vi "Build DashBoard Data.vi"() -> ()   [LabVIEW 2011]
doc: "This VI builds data and sends it back to the dashboard PC program. By default it sends back the raw values for the first analog, digital, and solenoid module. Modify it to send back the data you want to view. Consider adding higher level data to the Dashboard Datatype.ctl and to this VI. Then update the Dashboard to display the data however you like.\n\nThis software is licensed. Open the labview\\readme\\WPI Robotics Library Open Source License.txt file for more information."
uses:
  hiPri Dashboard Datatype.ctl
  Dashboard Datatype.ctl
  Robot Global Data.vi
panel:
  in  "Dashboard Data":T1={"Bridge Balance"=FALSE, "Gyro"=0.0, "Left Drive"=0.0, "Right Drive"=0.0, "Shooter Ready"=FALSE, "Compass"=0.0, "Turret Enc"=0.0, "Gear"=0, "Turret Postion"=1.0, "Turret Bump"=FALSE, "Collector System Enabled?"=FALSE, "Personality"="", "Brake"=FALSE} {"Gear" items=["HIGH", "LOW"]; "Compass" scale=0.0..-180.0; "Gyro" scale=-180.0..180.0}
  in  "HiPri":T2
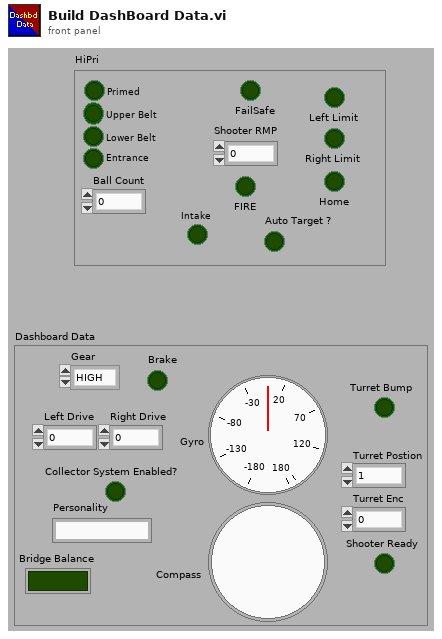
[diagram p1: front panel]
types:
  T1 = typedef "Dashboard Datatype.ctl" = cluster{"Bridge Balance":bool, "Gyro":dbl, "Left Drive":dbl, "Right Drive":dbl, "Shooter Ready":bool, "Compass":dbl, "Turret Enc":dbl, "Gear":u16, "Turret Postion":dbl, "Turret Bump":bool, "Collector System Enabled?":bool, "Personality":string, "Brake":bool}
  T2 = typedef "hiPri Dashboard Datatype.ctl" = cluster{"Ball Count":dbl, "Shooter RMP":dbl, "FIRE":bool, "FailSafe":bool, "Entrance":bool, "Lower Belt":bool, "Upper Belt":bool, "Primed":bool, "Intake":bool, "Right Limit":bool, "Home":bool, "Left Limit":bool, "Auto Target ?":bool}
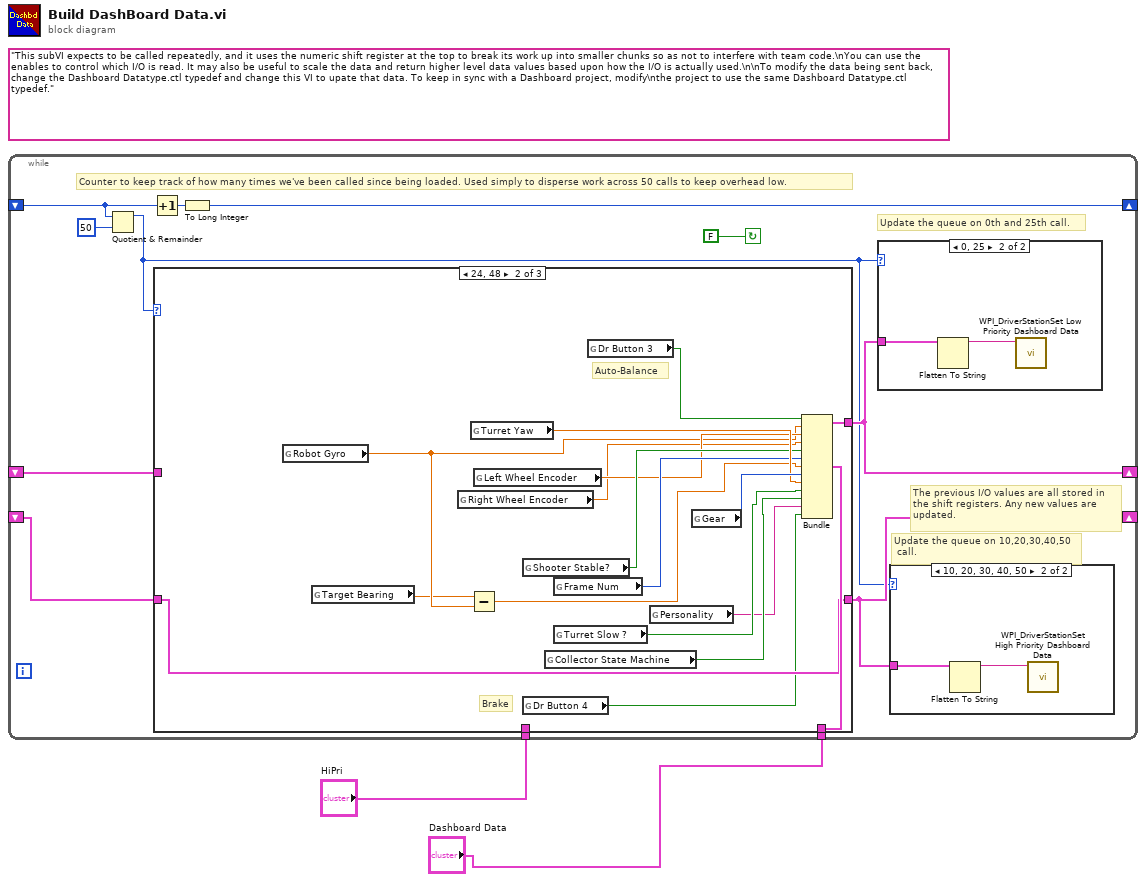
[diagram p0: block diagram]
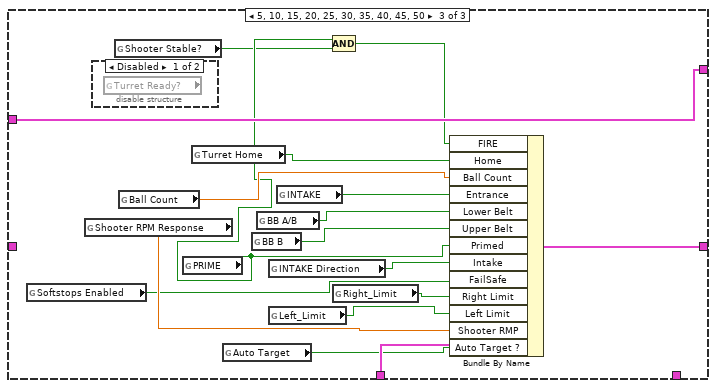
[diagram p5: hidden frame]
diagram:
  (unwired) "This subVI expects to be called repeatedly, and it uses the numeric shift register at the top to break its work up into smaller chunks so as not to interfere with team code.\nYou can use the enables to control which I/O is read. It may also be useful to scale the data and return higher level data values based upon how the I/O is actually used.\n\nTo modify the data being sent back, change the Dashboard Datatype.ctl typedef and change this VI to upate that data. To keep in sync with a Dashboard project, modify\nthe project to use the same Dashboard Datatype.ctl typedef."
  n1 = while {
    shift-right: [w9] -> _
    shift-left: _ -> [w10]
    shift-right: [w7] -> _
    shift-left: _ -> [w12]
    tunnel: "Dashboard Data" -> [w8]
    tunnel: "HiPri" -> [w6]
    shift-right: [w5] -> _
    shift-left: _ -> [w4]
    stop <- FALSE continue-if-true
    # "Update the queue on 10,20,30,40,50\n call."
    # "Counter to keep track of how many times we've been called since being loaded. Used simply to disperse work across 50 calls to keep overhead low."
    # "Update the queue on 0th and 25th call."
    # "The previous I/O values are all stored in\nthe shift registers. Any new values are\nupdated."
    n2 = Quotient & Remainder(x=w10, y=50) -> (x-y*floor(x/y)=w3:i32)  [unwired: 1 out]
    n3 = Increment(x=w10) -> (x+1=w14:i32)
    n4 = case shown="24, 48" w3 {
      tunnel: [w20 w36 w54] -> w7
      tunnel: w12 -> [w20 _ w54]
      tunnel: w8 -> [_ w37 _]
      tunnel: w6 -> [_ _ w53]
      tunnel: [w19 w35 w52] -> w5
      tunnel: w4 -> [w19 w35 _]
      frame Default {
        # "Don't update any I/O"
      }
      frame 24, 48 {
        # "Brake"
        # "Auto-Balance"
        n5 = global read "Robot Global Data.vi" "Robot Gyro"() -> (w26:dbl)
        n6 = global read "Robot Global Data.vi" "Target Bearing"() -> (w25:dbl)
        n7 = global read "Robot Global Data.vi" "Right Wheel Encoder"() -> (w29:dbl)
        n8 = Subtract(x=w25, y=w26) -> (x-y=w24:dbl)
        n9 = global read "Robot Global Data.vi" "Turret Yaw"() -> (w33:dbl)
        n10 = global read "Robot Global Data.vi" "Left Wheel Encoder"() -> (w30:dbl)
        n11 = global read "Robot Global Data.vi" "Shooter Stable?"() -> (w31:bool)
        n12 = global read "Robot Global Data.vi" "Dr Button 4"() -> (w21:bool)
        n13 = global read "Robot Global Data.vi" "Collector State Machine"() -> (w27:bool)
        n14 = global read "Robot Global Data.vi" "Frame Num"() -> (w32:i32)
        n15 = global read "Robot Global Data.vi" "Turret Slow ?"() -> (w28:bool)
        n16 = global read "Robot Global Data.vi" "Dr Button 3"() -> (w22:bool)
        n17 = global read "Robot Global Data.vi" "Personality"() -> (w23:string)
        n18 = global read "Robot Global Data.vi" "Gear"() -> (w34:u16)
        n19 = Bundle(cluster=w37, "Bridge Balance"=w22, "Gyro"=w26, "Left Drive"=w30, "Right Drive"=w29, "Shooter Ready"=w31, "Compass"=w32, "Turret Enc"=w24, "Gear"=w34, "Turret Postion"=w33, "Turret Bump"=w28, "Collector System Enabled?"=w27, "Personality"=w23, "Brake"=w21) -> (w36:T1)
      }
      frame 5, 10, 15, 20, 25, 30, 35, 40, 45, 50 {
        n20 = global read "Robot Global Data.vi" "Softstops Enabled"() -> (w45:bool)
        n21 = global read "Robot Global Data.vi" "Shooter RPM Response"() -> (w50:dbl)
        n22 = disable-structure shown="Disabled" {
          frame Disabled {
            n23 = global read "Robot Global Data.vi" "Turret Ready?"() -> ()  [unwired: 1 out]
          }
          frame Enabled {
          }
        }
        n24 = global read "Robot Global Data.vi" "Shooter Stable?"() -> (w38:bool)
        n25 = global read "Robot Global Data.vi" "Ball Count"() -> (w49:dbl)
        n26 = global read "Robot Global Data.vi" "PRIME"() -> (w43:bool)
        n27 = global read "Robot Global Data.vi" "Turret Home"() -> (w51:bool)
        n28 = global read "Robot Global Data.vi" "Auto Target"() -> (w39:bool)
        n29 = global read "Robot Global Data.vi" "BB B"() -> (w46:bool)
        n30 = global read "Robot Global Data.vi" "BB A/B"() -> (w47:bool)
        n31 = global read "Robot Global Data.vi" "INTAKE Direction"() -> (w44:bool)
        n32 = global read "Robot Global Data.vi" "Left_Limit"() -> (w40:bool)
        n33 = global read "Robot Global Data.vi" "INTAKE"() -> (w48:bool)
        n34 = Compound Arithmetic op=AND(w43, w38) -> (w42:bool)
        n35 = global read "Robot Global Data.vi" "Right_Limit"() -> (w41:bool)
        n36 = Bundle By Name(cluster=w53, "FIRE"=w42, "Home"=w51, "Ball Count"=w49, "Entrance"=w48, "Lower Belt"=w47, "Upper Belt"=w46, "Primed"=w43, "Intake"=w44, "FailSafe"=w45, "Right Limit"=w41, "Left Limit"=w40, "Shooter RMP"=w50, "Auto Target ?"=w39) -> (w52:T2)
      }
    }
    n37 = To Long Integer(number=w14) -> (32bit integer=w9:i32)
    n38 = case shown="0, 25" w3 {
      tunnel: w7 -> [_ w18]
      frame Default {
      }
      frame 0, 25 {
        n39 = Flatten To String(anything=w18) -> (data string=w17:string)  [unwired: 1 in, 4 out]
        n40 = call <vilib>:"WPI_DriverStationSet Low Priority Dashboard Data.vi"("User Data"=w17) -> ()  [unwired: 1 in, 10 out]
      }
    }
    n41 = case shown="10, 20, 30, 40, 50" w3 {
      tunnel: w5 -> [_ w16]
      frame Default {
      }
      frame 10, 20, 30, 40, 50 {
        n42 = Flatten To String(anything=w16) -> (data string=w15:string)  [unwired: 1 in, 4 out]
        n43 = call <vilib>:"WPI_DriverStationSet High Priority Dashboard Data.vi"("User Data"=w15) -> ()  [unwired: 10 in, 1 out]
      }
    }
  }
